vi "counts_to_voltages.vi"(1 "Count Array":i16[][](array[numeric])) -> (0 "Voltage Array":dbl[][](array[numeric]))   [LabVIEW 2014]
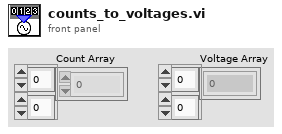
[diagram p1: front panel]
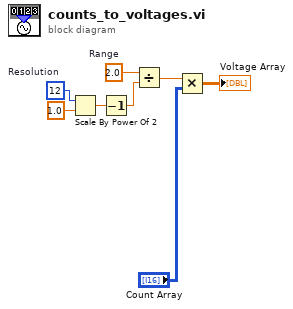
[diagram p0: block diagram]
diagram:
  w3 = 12  # Resolution
  w5 = 2.0  # Range
  n1 = Scale By Power Of 2(n=w3, x=1.0) -> (x*2^n=w2:dbl)
  n2 = Decrement(x=w2) -> (x-1=w1:dbl)
  n3 = Divide(x=w5, y=w1) -> (x/y=w6:dbl)
  n4 = Multiply(x=w6, y="Count Array") -> (x*y=→"Voltage Array":dbl[][])
